vi "Verify Cooler.vi"(8 "error in (no error)":errorcluster, 11 "Cooler.lvclass":refnum<class "Cooler.lvclass">) -> (0 "error out":errorcluster, 2 "coolerStatus":bool, 3 "Cooler.lvclass":refnum<class "Cooler.lvclass">)   [LabVIEW 2018, in "Cooler.lvclass"]
doc: "Este VI verifica se o cooler está ligado."
uses:
  Cooler.lvclass
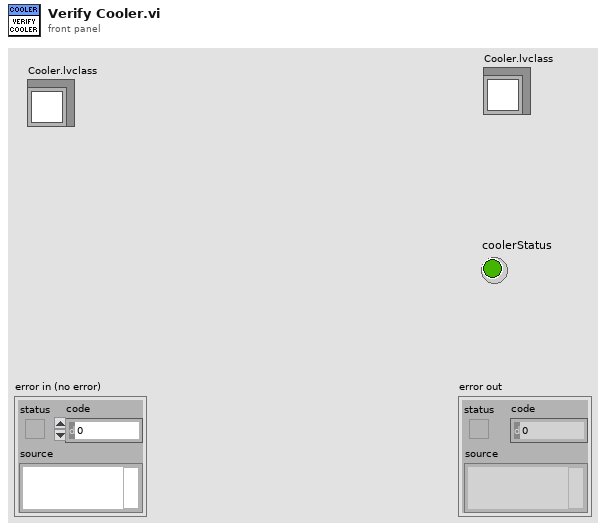
[diagram p1: front panel]
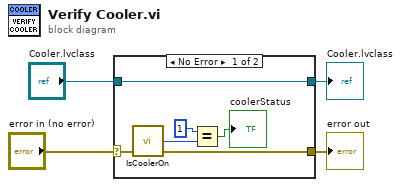
[diagram p0: block diagram]
diagram:
  n1 = case shown="No Error" "error in (no error)" {
    selector: "error in (no error)" -> [w10 w12]
    tunnel: [w9 w12] -> w3
    tunnel: [w5 w11] -> w1
    tunnel: "Cooler.lvclass" -> [w5 w11]
    frame No Error {
      n2 = call <userlib>:"IsCoolerOn.vi"("error in (no error)"=w10) -> ("error out"=w9:errorcluster, "coolerStatus"=w8:i32)  [unwired: 2 in, 1 out]
      n3 = Equal?(x=1, y=w8) -> (x = y?=→"coolerStatus":bool)
    }
    frame Error {
    }
  }
  "error out" <- w3
  "Cooler.lvclass" <- w1
